vi "RT - Create Or Write Config File.vi"(8 "error in":errorcluster, 9 "CONFIG DATA":T2={"PDP (IN)"=[1.0, 2.2, 1.0, 1.744, 1.4, 5.3, 0.873, 8.975], "SETTINGS"=[100.0, 500.0, 200.0, 2800.0, 30.0, 180.0], "TIMEOUTS (SEC)"=[20.0, 20.0, 60.0, 20.0, 20.0, 60.0, 20.0, 30.0, 60.0]}, 10 "CONFIG STRING":T1={"PDP (IN)"=["TWTT OP (IN)", "TWTT PDP (IN)", "DLT OP (IN)", "DLT PDP 01 (IN)", "DLT PDP 02 (IN)", "BR OP (IN)", "BR TWT ALIGN", "BR DL ALIGN (IN)"], "SETTINGS"=["HPL Low (PSI)", "HPL High (PSI)", "HPH Low (PSI)", "HPH High (PSI)", "AP Low (PSI)", "AP High (PSI)", "DL Clean (SEC)", "Reset (MIN)"], "TIMEOUTS (SEC)"=["TWTT Drive (SEC)", "DL Drive (SEC)", "DL Rotate (SEC)", "BR Drive (SEC)", "OT Engage (SEC)", "Plug Drive (SEC)", "IT Engage (SEC)", "IT 1REV (SEC)", "IT nREV (SEC)"]}, 11 "ConfigFile Path In":path) -> (0 "error out":errorcluster, 3 "ConfigFile Path Out":path)   [LabVIEW 2018]
uses:
  Controls/ConfigData.ctl
  Controls/ConfigString.ctl
  <vilib>/Utility/config.llb/Write Key (Double).vi
  <vilib>/Utility/config.llb/NI_LVConfig.lvlib
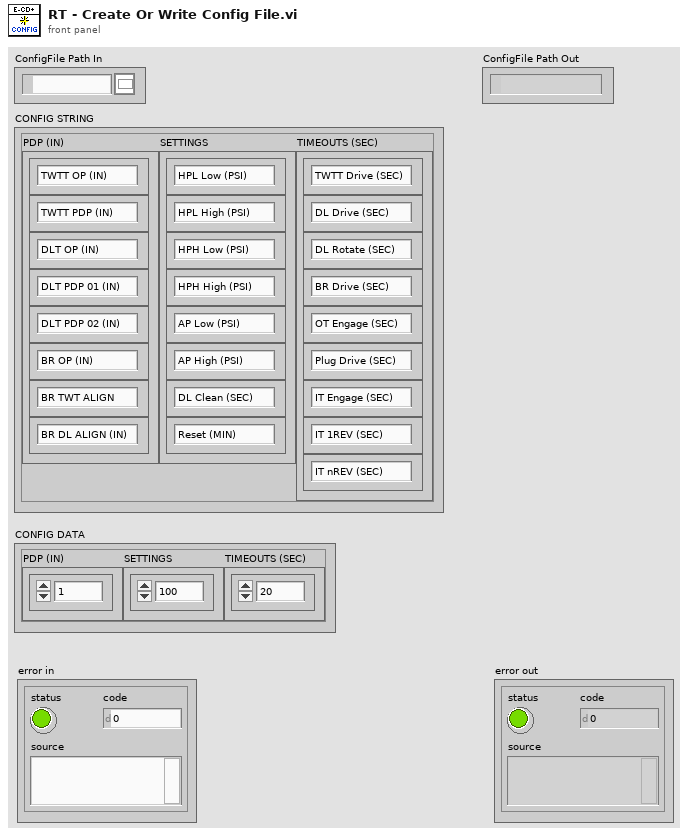
[diagram p1: front panel]
types:
  T1 = typedef "ConfigString.ctl" = cluster{"PDP (IN)":string[], "SETTINGS":string[], "TIMEOUTS (SEC)":string[]}
  T2 = typedef "ConfigData.ctl" = cluster{"PDP (IN)":dbl[], "SETTINGS":dbl[], "TIMEOUTS (SEC)":dbl[]}
  T3 = typedef "NI_LVConfig.lvlib/Config Data RefNum.ctl" = refnum<k1>
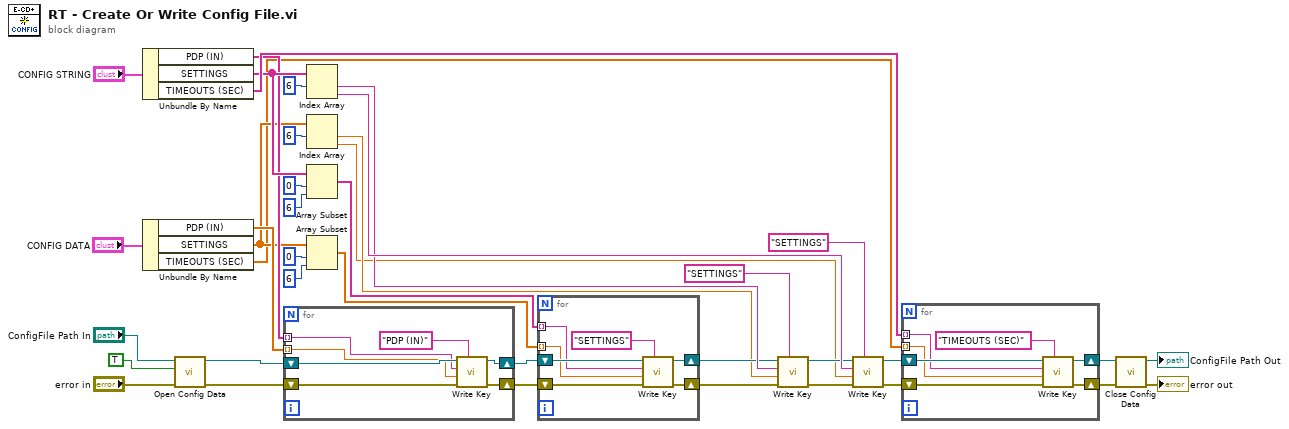
[diagram p0: block diagram]
diagram:
  n1 = Unbundle By Name("CONFIG STRING") -> ("PDP (IN)"=w37:string[], "SETTINGS"=w38:string[], "TIMEOUTS (SEC)"=w39:string[])
  n2 = Unbundle By Name("CONFIG DATA") -> ("PDP (IN)"=w10:dbl[], "SETTINGS"=w5:dbl[], "TIMEOUTS (SEC)"=w2:dbl[])
  n3 = call <vilib>:"Open Config Data.vi"("error in (no error)"="error in", "create file if necessary (T)"=TRUE, "configuration file path"="ConfigFile Path In") -> ("error out"=w14:errorcluster, "refnum"=w15:T3)  [unwired: 6 in, 1 out]
  n4 = for {
    shift-right: [w45] -> w16
    shift-left: w14 -> [w46]
    shift-right: [w43] -> w17
    shift-left: w15 -> [w44]
    tunnel: w37 -> [w42] mode=indexing
    tunnel: w10 -> [w41] mode=indexing
    n5 = call-poly <vilib>:"Write Key.vi"("section"="PDP (IN)", "error in (no error)"=w46, "value"=w41, "key"=w42, "refnum"=w44) -> ("error out"=w45:errorcluster, "refnum out"=w43:T3)  [unwired: 4 in, 1 out]
  }
  n6 = Index Array(array=w38, index #1=6 ("index")) -> (element #1=w35:string, element #2=w36:string)  [unwired: 1 in]
  n7 = Index Array(array=w5, index #1=6 ("index")) -> (element #1=w4:dbl, element #2=w3:dbl)  [unwired: 1 in]
  n8 = Array Subset(array=w38, index=0, length=6) -> (w33:string[])
  n9 = Array Subset(array=w5, index=0, length=6) -> (w7:dbl[])
  n10 = for {
    shift-right: [w52] -> w22
    shift-left: w16 -> [w53]
    shift-right: [w50] -> w19
    shift-left: w17 -> [w51]
    tunnel: w33 -> [w49] mode=indexing
    tunnel: w7 -> [w47] mode=indexing
    n11 = call-poly <vilib>:"Write Key.vi"("section"="SETTINGS", "error in (no error)"=w53, "value"=w47, "key"=w49, "refnum"=w51) -> ("error out"=w52:errorcluster, "refnum out"=w50:T3)  [unwired: 4 in, 1 out]
  }
  n12 = call-poly <vilib>:"Write Key.vi"("section"="SETTINGS", "error in (no error)"=w22, "value"=w4, "key"=w35, "refnum"=w19) -> ("error out"=w23:errorcluster, "refnum out"=w21:T3)  [unwired: 4 in, 1 out]
  n13 = call-poly <vilib>:"Write Key.vi"("section"="SETTINGS", "error in (no error)"=w23, "value"=w3, "key"=w36, "refnum"=w21) -> ("error out"=w25:errorcluster, "refnum out"=w24:T3)  [unwired: 4 in, 1 out]
  n14 = for {
    shift-right: [w59] -> w26
    shift-left: w25 -> [w60]
    shift-right: [w57] -> w27
    shift-left: w24 -> [w58]
    tunnel: w39 -> [w55] mode=indexing
    tunnel: w2 -> [w54] mode=indexing
    n15 = call-poly <vilib>:"Write Key.vi"("section"="TIMEOUTS (SEC)", "error in (no error)"=w60, "value"=w54, "key"=w55, "refnum"=w58) -> ("error out"=w59:errorcluster, "refnum out"=w57:T3)  [unwired: 4 in, 1 out]
  }
  n16 = call <vilib>:"Close Config Data.vi"("error in (no error)"=w26, "refnum"=w27) -> ("error out"=→"error out":errorcluster, "file path"=→"ConfigFile Path Out":path)  [unwired: 1 in, 7 out]
